vi "Node_Adjust.vi"(1 "PicAjust":T1={"TranslationVector"=[], "scale"=1.0, "Pitch（x) "=0.0, "Yaw（y)"=0.0, "Roll（z) "=0.0} {"Roll（z)" scale=-90.0..90.0; "Yaw（y)" scale=-90.0..90.0; "Pitch（x)" scale=-90.0..90.0}, 2 "Node":dbl[](array[numeric])=[50.0, 50.0, 500.0], 3 "视图":enum16{"俯视图", "轴测图"}(ring)) -> (0 "NewNode":dbl[](array[numeric]))   [LabVIEW 2014]
doc: "实现俯视图和轴测图切换"
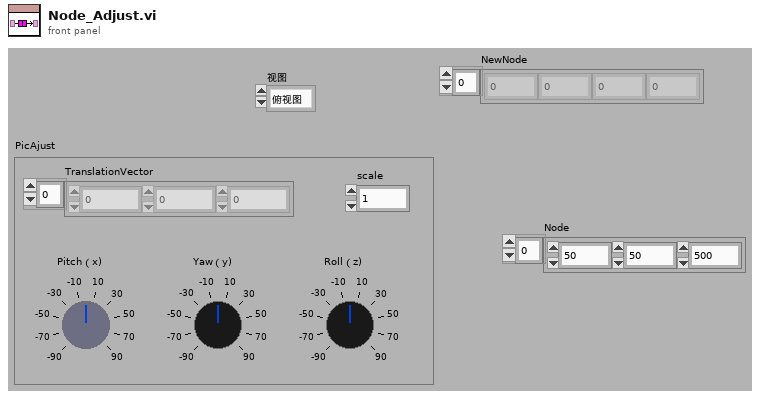
[diagram p1: front panel]
types:
  T1 = cluster{"TranslationVector":dbl[], "scale":dbl, "Pitch（x) ":dbl, "Yaw（y)":dbl, "Roll（z) ":dbl}
  T2 = typedef "NI_Kinematics.lvlib/Quaternion.ctl" = dbl[]
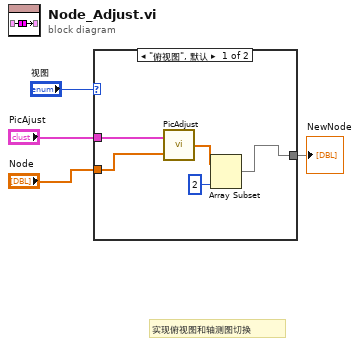
[diagram p0: block diagram]
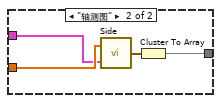
[diagram p2: hidden frame]
diagram:
  # "实现俯视图和轴测图切换"
  n1 = case shown="\"俯视图\", 默认" "视图" {
    tunnel: "Node" -> [w8 w13]
    tunnel: "PicAjust" -> [w9 w12]
    tunnel: [w7 w11] -> w1
    frame "俯视图", Default {
      n2 = call "PicAdjust.vi"("Input"=w8, "PicAjust"=w9) -> ("子数组"=w6:T2)
      n3 = Array Subset(array=w6, length=2 ("长度")) -> (w7:T2)  [unwired: 1 in]
    }
    frame "轴测图" {
      n4 = call "Side.vi"("PicAjust"=w12, "Input"=w13) -> ("输出簇"=w10:cluster{"x":dbl, "y":dbl})
      n5 = Cluster To Array(cluster=w10) -> (array=w11:dbl[])
    }
  }
  "NewNode" <- w1
